vi "Fetch Room Size Details.vi"(0 "File Data Manager in":refnum<class "File Data Manager.lvclass">, 5 "Room No":string, 11 "error in (no error)":errorcluster) -> (4 "File Data Manager out":refnum<class "File Data Manager.lvclass">, 6 "Room Size Details":T1, 15 "error out":errorcluster)   [LabVIEW 2023, in "File Data Manager.lvlib" / "File Data Manager.lvclass"]
uses:
  File Data Manager.lvclass
  File Data Manager.lvclass/File Data Manager.ctl
  Central Data Manager/Central Data Manager/Central Data Manager.lvclass
  Central Data Manager/Central Data Manager/Room Size Details.ctl
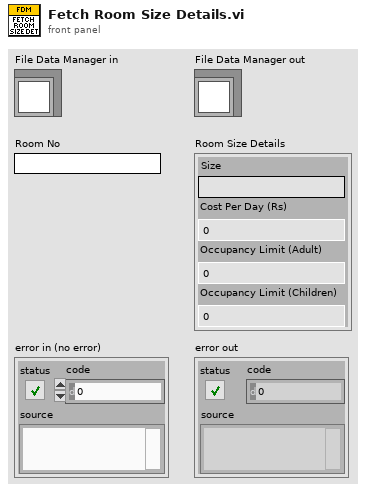
[diagram p1: front panel]
types:
  T1 = typedef "Central Data Manager.lvlib/Central Data Manager.lvclass/Room Size Details.ctl" = cluster{"Size":string, "Cost Per Day (Rs)":u32, "Occupancy Limit (Adult)":u32, "Occupancy Limit (Children)":u32}
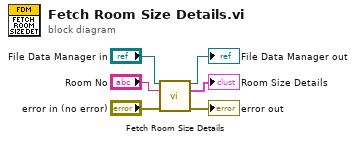
[diagram p0: block diagram]
diagram:
  n1 = call-parent "Fetch Room Size Details.vi"("Central Data Manager in"="File Data Manager in", "Room No"="Room No", "error in (no error)"="error in (no error)") -> ("Central Data Manager out"=→"File Data Manager out":refnum<class "File Data Manager.lvclass">, "Room Size Details"=→"Room Size Details":T1, "error out"=→"error out":errorcluster)  [unwired: 10 in]
